vi "Disconnect.vi"(8 "error in":errorcluster, 11 "FPGA-DIO in":refnum<class "FPGA_DIO.lvclass">) -> (0 "error out":errorcluster, 3 "FPGA-DIO out":refnum<class "FPGA_DIO.lvclass">)   [LabVIEW 2019, in "FPGA_DIO.lvlib" / "FPGA_DIO.lvclass"]
doc: "This override VI is a carryover override from the parent class, children classes *must* override this VI and therefore the parent class must contain this VI to maintain the override rules."
uses:
  Library/FPGA_DIO.lvclass
  builds/Instruments/DIG_IO.lvlibp/Library/DIG_IO.lvclass
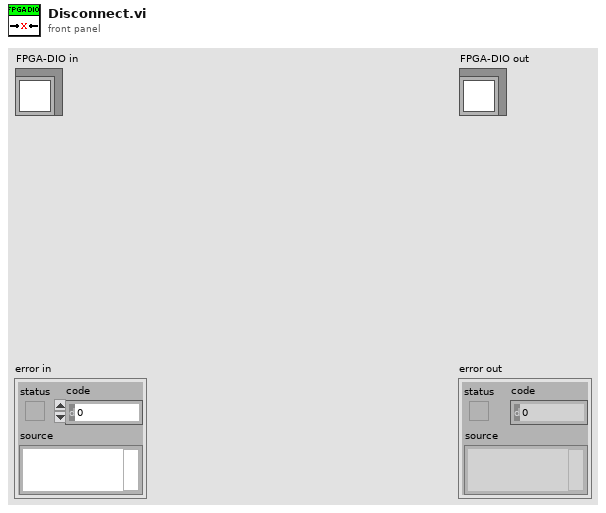
[diagram p1: front panel]
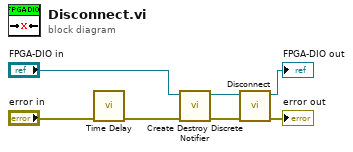
[diagram p0: block diagram]
diagram:
  n1 = call "Time Delay"("error in (no error)"="error in") -> ("error out"=w1:errorcluster)  [unwired: 10 in]
  n2 = call "Create Destroy Discrete Notifier.vi"("error in"=w1, "FPGA-DIO in"="FPGA-DIO in") -> ("error out"=w3:errorcluster, "FPGA-DIO out"=w2:refnum<class "FPGA_DIO.lvclass">)  [unwired: 8 in]
  n3 = call-parent "Disconnect.vi"("error in"=w3, "DIG_IO in"=w2) -> ("error out"=→"error out":errorcluster, "DIG_IO out"=→"FPGA-DIO out":refnum<class "FPGA_DIO.lvclass">)  [unwired: 8 in]
